vi "Subscribe to Did Initiailze.vi"(8 "error in (no error)":errorcluster, 11 "API-Reference in":refnum<data-value>) -> (0 "error out":errorcluster, 2 "Event Registration Refnum":refnum<event-registration>, 3 "API-Reference out":refnum<data-value>)   [LabVIEW 2018, in "Templates.lvlib" / "Actor.lvclass"]
uses:
  Actor.lvclass
  API-Data.ctl
  Did Stop.ctl
  Message-Enqueuer References.ctl
  Stop.ctl
  Launch.ctl
  Did Initialize.ctl
  Did Initialize Reference.ctl
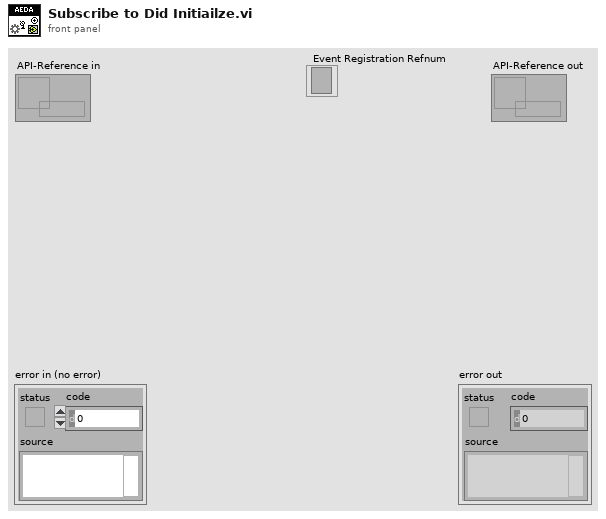
[diagram p1: front panel]
types:
  T1 = typedef "Templates.lvlib/Actor.lvclass/API-Data.ctl" = cluster{"Launch":refnum<notifier>, "Did Stop Enqueuer":refnum<user-event>, "API":T2, "Did Stop Messages":refnum<event-registration>}
  T2 = typedef "Templates.lvlib/Actor.lvclass/Message-Enqueuer References.ctl" = cluster{"Stop":refnum<user-event>, "Launch":refnum<user-event>, "Did Initialize":refnum<user-event>}
  T3 = typedef "Templates.lvlib/Actor.lvclass/Did Initialize Reference.ctl" = refnum<user-event>
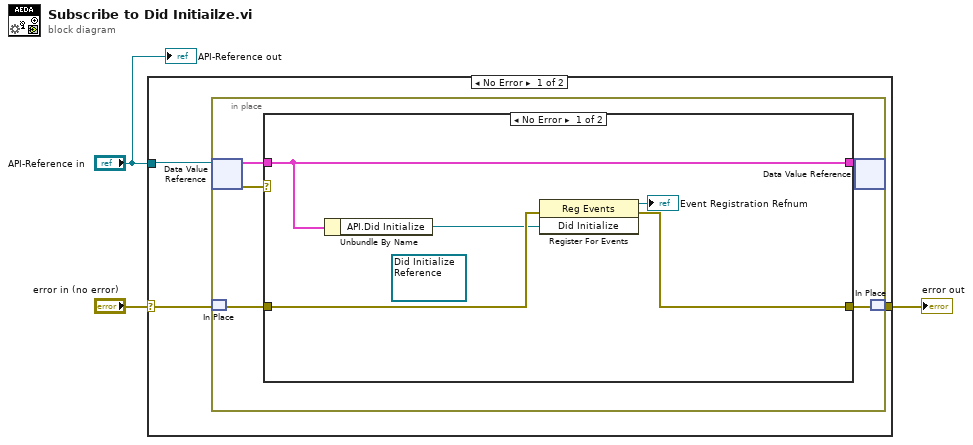
[diagram p0: block diagram]
diagram:
  n1 = case shown="No Error" "error in (no error)" {
    selector: "error in (no error)" -> [w6 w19]
    tunnel: [w5 w19] -> w2
    tunnel: "API-Reference in" -> [w4 _]
    frame No Error {
      n2 = in-place {
        n3 = in-place-dvr #1(w4) -> (w10:T1, w11:errorcluster)
        n4 = in-place-match #2(w6) -> (w8:errorcluster)
        n5 = case shown="No Error" w11 {
          selector: w11 -> [_ w18]
          tunnel: w10 -> [w13 w17]
          tunnel: [w13 w17] -> w9
          tunnel: w8 -> [w16 _]
          tunnel: [w15 w18] -> w7
          frame No Error {
            (unwired) T3 refnum ("Message Enqueuers.Did Initialize")
            n6 = Unbundle By Name(w13) -> ("API.Did Initialize"=w14:refnum<user-event>)
            n7 = register-events(error in=w16, w14) -> (reference out=→"Event Registration Refnum":refnum<event-registration>, error out=w15:errorcluster)  [unwired: 1 in]
          }
          frame Error {
          }
        }
        n8 = in-place-dvr #1(w9) -> ()  [unwired: 2 out]
        n9 = in-place-match #2(w7) -> (w5:errorcluster)
      }
    }
    frame Error {
    }
  }
  "error out" <- w2
  "API-Reference out" <- "API-Reference in"
